vi "Security.FG.vi"(7 "Action":T1, 8 "error in (no error)":errorcluster, 10 "Security":T2={"Type"=enum."None", "Source DLL Path"=path "", "Target DLL Path"=path "", "Security Level"=1, "Static Master Key"="", "Max Key Length"=1, "Host IP Address"="", "ECU  Variant"=0, "Optional Parameter"=0}, 11 "Device Item Ref in":T4 format="%.0x") -> (0 "error out":errorcluster, 2 "Security":T2={"Type"=enum."None", "Source DLL Path"=path "", "Target DLL Path"=path "", "Security Level"=1, "Static Master Key"="", "Max Key Length"=1, "Host IP Address"="", "ECU  Variant"=0, "Optional Parameter"=0}, 3 "Device Item Ref out":T4=18446744073709551615 format="%.0x")   [LabVIEW 2019, in "Diagnostics Addon System Explorer.lvlib"]
uses:
  Diagnostics Addon System Explorer.lvlib
  <vilib>/NI VeriStand/Custom Device API/Custom Device Item Ref.ctl
  Addon Shared/Types/Security.ctl
  Addon Shared/Types/Security.Type.ctl
  Types/FG.Action.ctl
  Addon Shared/SubVIs/Constants.vi
  <vilib>/NI VeriStand/Custom Device API/Get Item Property (U32).vi
  <vilib>/NI VeriStand/Custom Device API/Get Item Property (Path).vi
  <vilib>/NI VeriStand/Custom Device API/Get Item Property (Variant).vi
  <vilib>/NI VeriStand/Custom Device API/Get Item Property (String).vi
  <vilib>/NI VeriStand/Custom Device API/Get Item Property (I32).vi
  <vilib>/NI/NI VeriStand Advanced SysDef API/_SubVIs/SysDef.Property.Set.Path.vi
  <vilib>/Utility/MD5Checksum.llb/MD5Checksum File.vi
  <vilib>/NI/NI VeriStand Advanced SysDef API/_SubVIs/SysDef.Property.Set.DependentFile.vi
  <vilib>/NI/NI VeriStand Advanced SysDef API/_SubVIs/SysDef.Property.Set.U32.vi
  <vilib>/NI/NI VeriStand Advanced SysDef API/_SubVIs/SysDef.Property.Set.Variant.vi
  <vilib>/NI/NI VeriStand Advanced SysDef API/_SubVIs/SysDef.Property.Set.String.vi
  <vilib>/NI/NI VeriStand Advanced SysDef API/_SubVIs/SysDef.Property.Set.I32.vi
  Addon Shared/Diagnostics Addon Shared.lvlib
  <vilib>/NI VeriStand/Custom Device API/Custom Device API.lvlib
  <vilib>/NI/NI VeriStand Advanced SysDef API/SysDef API/Advanced System Definition.lvlib
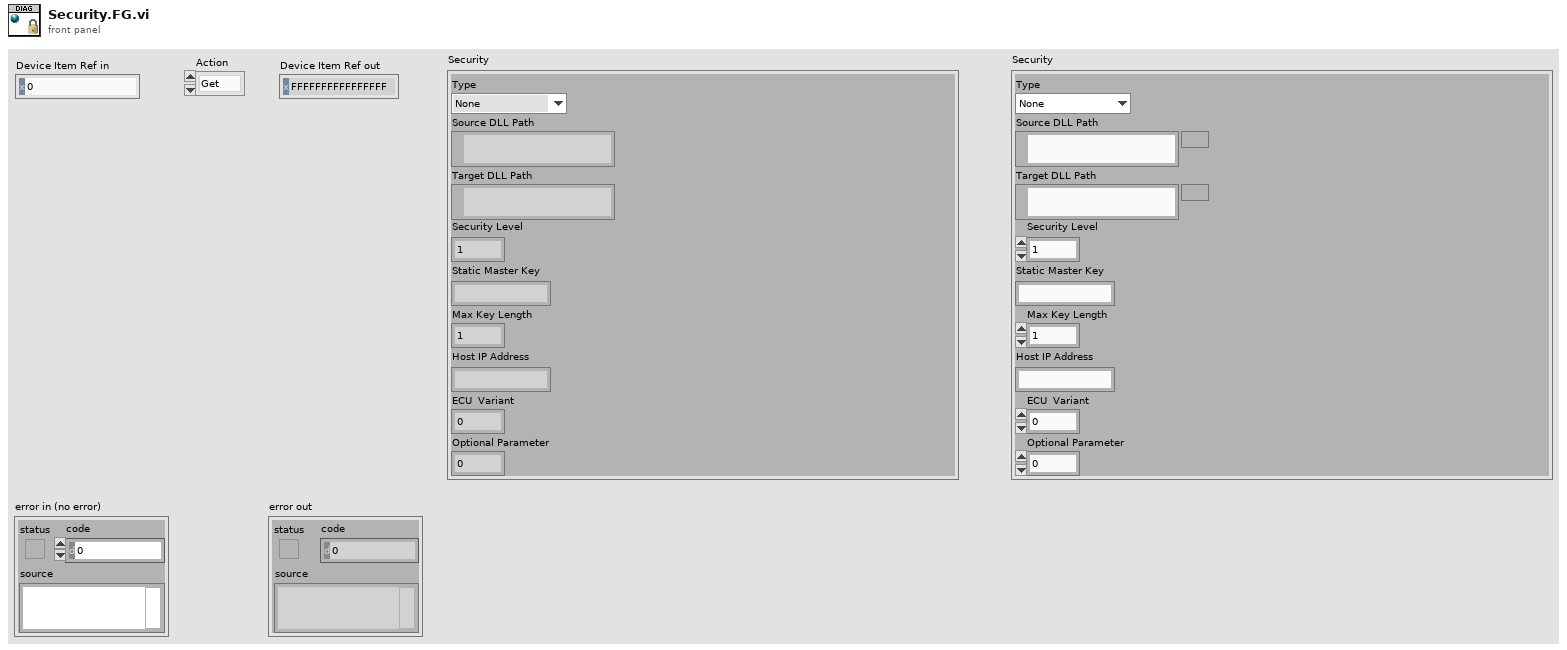
[diagram p1: front panel]
types:
  T1 = typedef "Diagnostics Addon System Explorer.lvlib/FG.Action.ctl" = enum16{"Get", "Set"}
  T2 = typedef "Diagnostics Addon Shared.lvlib/Security.ctl" = cluster{"Type":T3, "Source DLL Path":path, "Target DLL Path":path, "Security Level":u32, "Static Master Key":string, "Max Key Length":u32, "Host IP Address":string, "ECU  Variant":i8, "Optional Parameter":i8}
  T3 = typedef "Diagnostics Addon Shared.lvlib/Security.Type.ctl" = enum16{"None", "SeedKey DLL", "MasterKey (Channel)", "MasterKey (Static)", "SeedKey DLL (Windows)"}
  T4 = typedef "Custom Device API.lvlib/Custom Device Item Ref.ctl" = u64
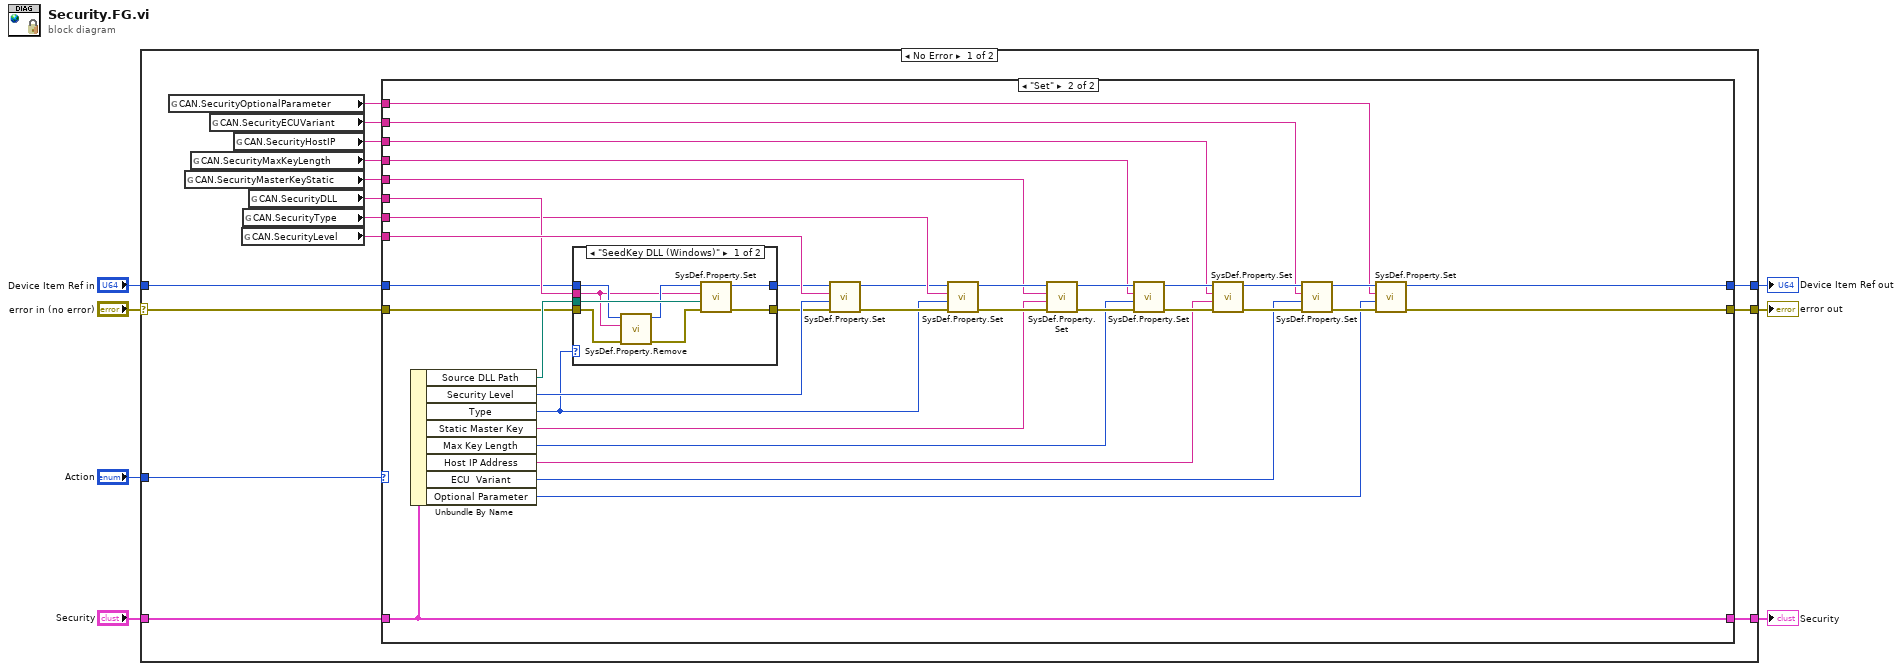
[diagram p0: block diagram]
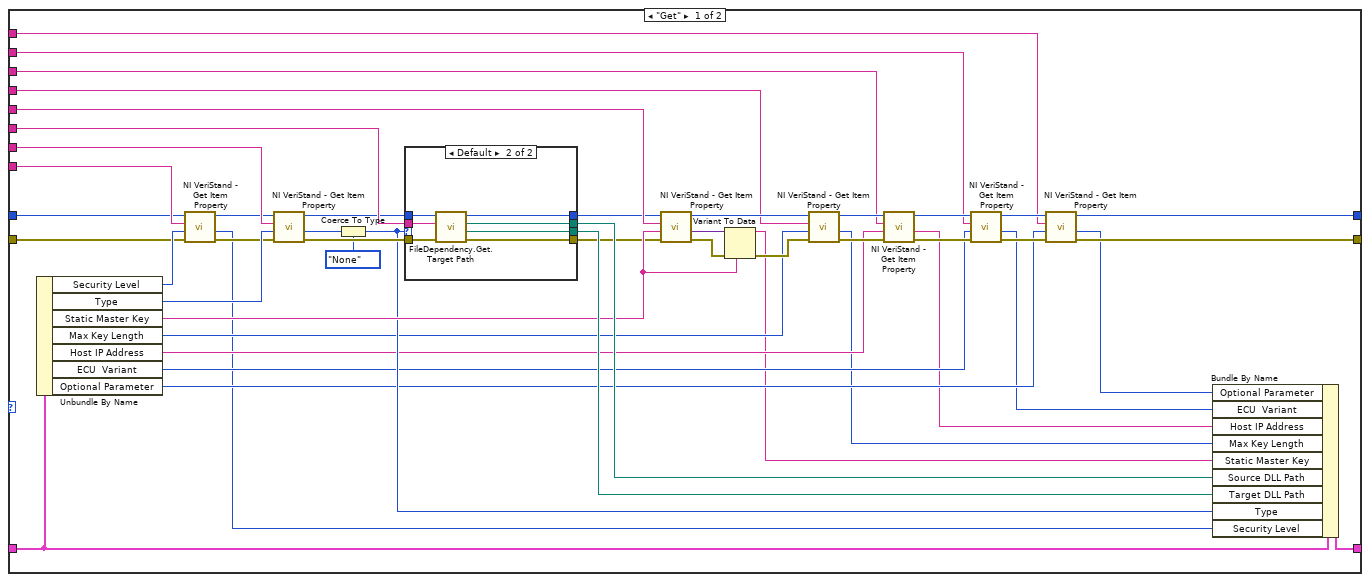
[diagram p2: hidden frame]
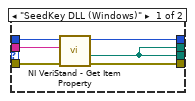
[diagram p3: hidden frame]
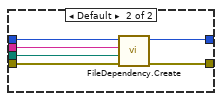
[diagram p4: hidden frame]
diagram:
  n1 = case shown="No Error" "error in (no error)" {
    selector: "error in (no error)" -> [w22 w133]
    tunnel: "Device Item Ref in" -> [w21 w134]
    tunnel: [w13 w134] -> w4
    tunnel: [w14 w133] -> w5
    tunnel: [w20 _] -> w3
    tunnel: "Security" -> [w19 _]
    tunnel: "Action" -> [w18 _]
    frame No Error {
      n2 = global read "Constants.vi" "CAN.SecurityOptionalParameter"() -> (w8:string)
      n3 = global read "Constants.vi" "CAN.SecurityMasterKeyStatic"() -> (w12:string)
      n4 = global read "Constants.vi" "CAN.SecurityMaxKeyLength"() -> (w11:string)
      n5 = global read "Constants.vi" "CAN.SecurityECUVariant"() -> (w9:string)
      n6 = global read "Constants.vi" "CAN.SecurityHostIP"() -> (w10:string)
      n7 = global read "Constants.vi" "CAN.SecurityLevel"() -> (w16:string)
      n8 = global read "Constants.vi" "CAN.SecurityType"() -> (w15:string)
      n9 = global read "Constants.vi" "CAN.SecurityDLL"() -> (w17:string)
      n10 = case shown="\"Set\"" w18 {
        tunnel: w22 -> [w55 w109]
        tunnel: w21 -> [w54 w110]
        tunnel: [w69 w118] -> w20
        tunnel: w19 -> [w70 w118]
        tunnel: w17 -> [w66 w113]
        tunnel: w16 -> [w67 w116]
        tunnel: w15 -> [w63 w111]
        tunnel: [w38 w93] -> w14
        tunnel: [w37 w92] -> w13
        tunnel: w12 -> [w59 w104]
        tunnel: w11 -> [w36 w87]
        tunnel: w10 -> [w35 w86]
        tunnel: w9 -> [w34 w85]
        tunnel: w8 -> [w33 w84]
        frame "Get" {
          n11 = Unbundle By Name(w70) -> ("Security Level"=w68:u32, "Type"=w62:T3, "Static Master Key"=w56:string, "Max Key Length"=w32:u32, "Host IP Address"=w31:string, "ECU  Variant"=w30:i8, "Optional Parameter"=w29:i8)
          n12 = call-poly <vilib>:"NI VeriStand - Get Item Property.vi"("error in (no error)"=w55, "Default Value"=w68, "Property Name"=w67, "Item Ref in"=w54) -> ("error out"=w61:errorcluster, "Value"=w23:u32, "Item Ref out"=w60:T4)  [unwired: 4 in, 1 out]
          n13 = call-poly <vilib>:"NI VeriStand - Get Item Property.vi"("error in (no error)"=w61, "Default Value"=w62, "Property Name"=w63, "Item Ref in"=w60) -> ("error out"=w51:errorcluster, "Value"=w48:u32, "Item Ref out"=w53:T4)  [unwired: 4 in, 1 out]
          n14 = Coerce To Type(0:w48, 1:Security.Type."None" ("Type")) -> (2:w47:T3)
          n15 = case shown="Default" w47 {
            tunnel: w66 -> [w74 w83]
            tunnel: [w73 w82] -> w65
            tunnel: [w73 w81] -> w64
            tunnel: w53 -> [w75 w80]
            tunnel: [w72 w79] -> w52
            tunnel: w51 -> [w76 w78]
            tunnel: [w71 w77] -> w50
            frame "SeedKey DLL (Windows)" {
              n16 = call-poly <vilib>:"NI VeriStand - Get Item Property.vi"("error in (no error)"=w76, "Property Name"=w74, "Item Ref in"=w75) -> ("error out"=w71:errorcluster, "Value"=w73:path, "Item Ref out"=w72:T4)  [unwired: 5 in, 1 out]
            }
            frame Default {
              n17 = call "FileDependency.Get.Target Path.vi"("error in (no error)"=w78, "Bitfile 986x"=w83, "Item Ref in"=w80) -> ("error out"=w77:errorcluster, "Target Path"=w82:path, "Source Path"=w81:path, "Item Ref out"=w79:T4)  [unwired: 5 in]
            }
          }
          n18 = call-poly <vilib>:"NI VeriStand - Get Item Property.vi"("error in (no error)"=w50, "Default Value"=w56, "Property Name"=w59, "Item Ref in"=w52) -> ("error out"=w57:errorcluster, "Value"=w58:variant, "Item Ref out"=w46:T4)  [unwired: 4 in, 1 out]
          n19 = Variant To Data(error in=w57, type=w56, Variant=w58) -> (data=w24:string, error out=w45:errorcluster)
          n20 = call-poly <vilib>:"NI VeriStand - Get Item Property.vi"("error in (no error)"=w45, "Default Value"=w32, "Property Name"=w36, "Item Ref in"=w46) -> ("error out"=w44:errorcluster, "Value"=w25:u32, "Item Ref out"=w43:T4)  [unwired: 4 in, 1 out]
          n21 = call-poly <vilib>:"NI VeriStand - Get Item Property.vi"("error in (no error)"=w44, "Default Value"=w31, "Property Name"=w35, "Item Ref in"=w43) -> ("error out"=w41:errorcluster, "Value"=w26:string, "Item Ref out"=w42:T4)  [unwired: 4 in, 1 out]
          n22 = call-poly <vilib>:"NI VeriStand - Get Item Property.vi"("error in (no error)"=w41, "Default Value"=w30, "Property Name"=w34, "Item Ref in"=w42) -> ("error out"=w39:errorcluster, "Value"=w27:i32, "Item Ref out"=w40:T4)  [unwired: 4 in, 1 out]
          n23 = call-poly <vilib>:"NI VeriStand - Get Item Property.vi"("error in (no error)"=w39, "Default Value"=w29, "Property Name"=w33, "Item Ref in"=w40) -> ("error out"=w38:errorcluster, "Value"=w28:i32, "Item Ref out"=w37:T4)  [unwired: 4 in, 1 out]
          n24 = Bundle By Name(cluster=w70, "Optional Parameter"=w28, "ECU  Variant"=w27, "Host IP Address"=w26, "Max Key Length"=w25, "Static Master Key"=w24, "Source DLL Path"=w64, "Target DLL Path"=w65, "Type"=w47, "Security Level"=w23) -> (w69:T2)
        }
        frame "Set" {
          n25 = Unbundle By Name(w118) -> ("Source DLL Path"=w112:path, "Security Level"=w117:u32, "Type"=w102:T3, "Static Master Key"=w103:string, "Max Key Length"=w91:u32, "Host IP Address"=w90:string, "ECU  Variant"=w89:i8, "Optional Parameter"=w88:i8)
          n26 = case shown="\"SeedKey DLL (Windows)\"" w102 {
            tunnel: [w125 w132] -> w115
            tunnel: [w126 w131] -> w114
            tunnel: w113 -> [w119 w129]
            tunnel: w112 -> [w124 w130]
            tunnel: w110 -> [w120 w127]
            tunnel: w109 -> [w122 w128]
            frame "SeedKey DLL (Windows)" {
              n27 = call <vilib>:"SysDef.Property.Remove.vi"("error in (no error)"=w122, "Property Name"=w119, "nodeID"=w120) -> ("error out"=w123:errorcluster, "nodeID out"=w121:u64)  [unwired: 6 in, 1 out]
              n28 = call-poly <vilib>:"SysDef.Property.Set.vi"("error in (no error)"=w123, "Value"=w124, "Property Name"=w119, "nodeID"=w121) -> ("error out"=w125:errorcluster, "nodeID out"=w126:u64)  [unwired: 6 in]
            }
            frame Default {
              n29 = call "FileDependency.Create.vi"("error in (no error)"=w128, "DLL Path"=w130, "DLL Property Name"=w129, "Item Ref in"=w127) -> ("error out"=w132:errorcluster, "Item Ref out"=w131:T4)  [unwired: 6 in]
            }
          }
          n30 = call-poly <vilib>:"SysDef.Property.Set.vi"("error in (no error)"=w115, "Value"=w117, "Property Name"=w116, "nodeID"=w114) -> ("error out"=w108:errorcluster, "nodeID out"=w107:u64)  [unwired: 6 in]
          n31 = call-poly <vilib>:"SysDef.Property.Set.vi"("error in (no error)"=w108, "Value"=w102, "Property Name"=w111, "nodeID"=w107) -> ("error out"=w106:errorcluster, "nodeID out"=w105:u64)  [unwired: 6 in]
          n32 = call-poly <vilib>:"SysDef.Property.Set.vi"("error in (no error)"=w106, "Value"=w103, "Property Name"=w104, "nodeID"=w105) -> ("error out"=w100:errorcluster, "nodeID out"=w101:u64)  [unwired: 6 in]
          n33 = call-poly <vilib>:"SysDef.Property.Set.vi"("error in (no error)"=w100, "Value"=w91, "Property Name"=w87, "nodeID"=w101) -> ("error out"=w98:errorcluster, "nodeID out"=w99:u64)  [unwired: 6 in]
          n34 = call-poly <vilib>:"SysDef.Property.Set.vi"("error in (no error)"=w98, "Value"=w90, "Property Name"=w86, "nodeID"=w99) -> ("error out"=w96:errorcluster, "nodeID out"=w97:u64)  [unwired: 6 in]
          n35 = call-poly <vilib>:"SysDef.Property.Set.vi"("error in (no error)"=w96, "Value"=w89, "Property Name"=w85, "nodeID"=w97) -> ("error out"=w94:errorcluster, "nodeID out"=w95:u64)  [unwired: 6 in]
          n36 = call-poly <vilib>:"SysDef.Property.Set.vi"("error in (no error)"=w94, "Value"=w88, "Property Name"=w84, "nodeID"=w95) -> ("error out"=w93:errorcluster, "nodeID out"=w92:u64)  [unwired: 6 in]
        }
      }
    }
    frame Error {
    }
  }
  "error out" <- w5
  "Device Item Ref out" <- w4
  "Security" <- w3
